vi "N9310A Sweep SR830 Record to file.vi"() -> ()   [LabVIEW 2018]
uses:
  <instrlib>/Stanford Research 830/Public/Data/Read (All Parameters).vi
  <instrlib>/Agilent N9310/Agilent N9310.lvlib
  <instrlib>/Stanford Research 830/Stanford Research 830.lvlib
panel:
  in  "File to save to":path
  out "Measured voltage (V, RMS)":dbl format="%#_6p"
  out "Measured frequency (Hz)":dbl format="%#_6p"
  in  "Input coupling":u16(ring) items=["AC", "DC"]
  in  "Input connection":u16(ring) items=["Single-Ended Voltage", "Differential Voltage", "1 MOhm Current Gain", "100 MOhm Current Gain"]
  in  "Dynamic reserve":i16(ring)=2 items=["High Reserve"=0, "Normal"=1, "Low Noise"=2, "Auto Reserve"=-1]
  in  "Sensitivity":i16(ring)=26 items=["Auto Gain"=-1, "2 nV/fA"=0, "5 nV/fA"=1, "10 nV/fA"=2, "20 nV/fA"=3, "50 nV/fA"=4, "100 nV/fA"=5, "200 nV/fA"=6, "500 nV/fA"=7, "1 uV/pA"=8, "2 uV/pA"=9, "5 uV/pA"=10, "10 uV/pA"=11, "20 uV/pA"=12, "50 uV/pA"=13, "100 uV/pA"=14, "200 uV/pA"=15, "500 uV/pA"=16, "1 mV/nA"=17, "2 mV/nA"=18, "5 mV/nA"=19, "10 mV/nA"=20, "20 mV/nA"=21, "50 mV/nA"=22, "100 mV/nA"=23, "200 mV/nA"=24, "500 mV/mA"=25, "1 V/uA"=26]
  in  "VISA resource name of Stanford SR830":refnum<visa-resource-name>="GPIB0::9::INSTR"
  in  "VISA resource name of Agilent N9310A":refnum<visa-resource-name>="USB0::0x0957::0x2018::01151879::INSTR"
  in  "Wait before measuring (s)":dbl=0.1 format="%#_6p"
  out "Step":dbl format="%^#_6e"
  out "Frequency (Hz)":dbl format="%#_6p"
  in  "Steps":dbl=5.0 format="%^#_6e"
  in  "Amplitude (V)":dbl=0.5 format="%#_6p"
  in  "End frequency (Hz)":dbl=2500.0 format="%#_6p"
  in  "Start frequency (Hz)":dbl=500.0 format="%#_6p"
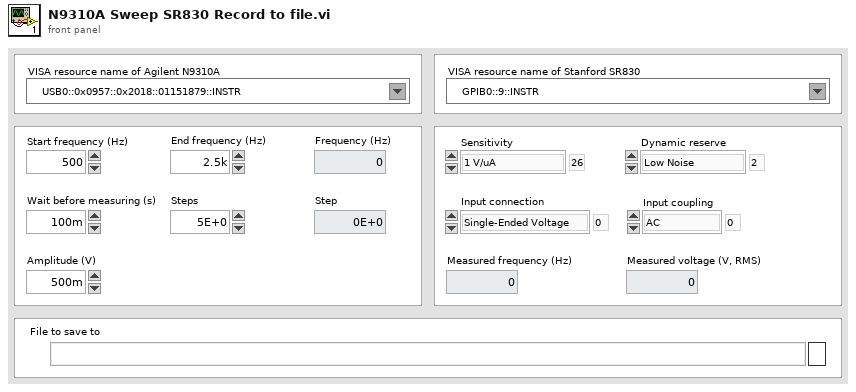
[diagram p1: front panel]
types:
  T1 = cluster{"X-Value":dbl, "Y-Value":dbl, "R-Value":dbl, "Theta-Value":dbl, "Aux In 1 Value":dbl, "Aux In 2 Value":dbl, "Aux In 3 Value":dbl, "Aux In 4 Value":dbl, "Reference Frequency":dbl, "Channel 1 Display":dbl, "Channel 2 Display":dbl}
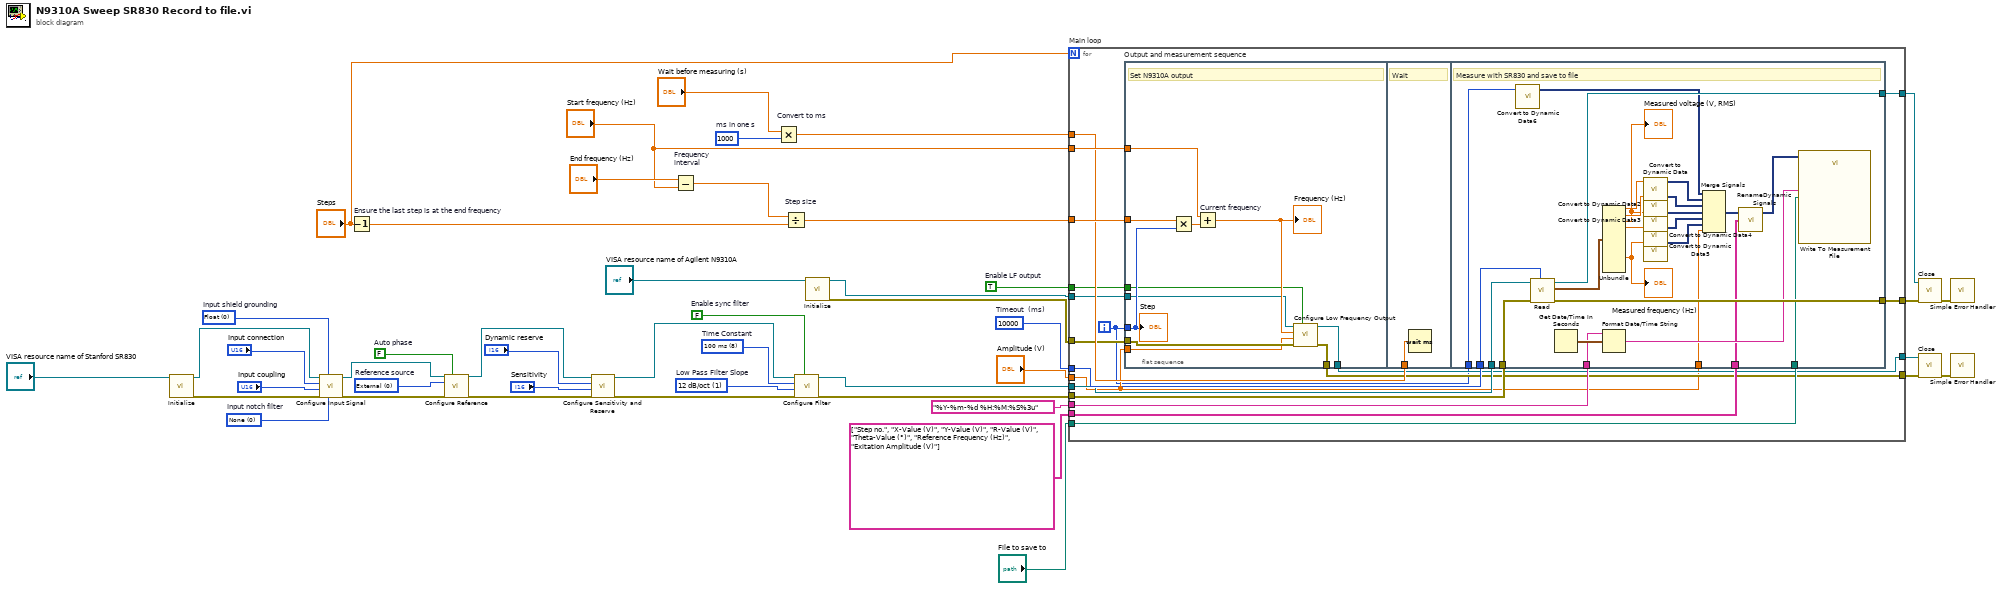
[diagram p0: block diagram]
diagram:
  w9 = u32 10000  # Timeout  (ms)
  w10 = u16 1 items=["6 dB/oct", "12 dB/oct", "18 db/oct", "24 dB/oct"]  # Low Pass Filter Slope
  w11 = u16 8 items=["10 us", "30 us", "100 us", "300 us", "1 ms", "3 ms", "10 ms", "30 ms", "100 ms", "300 ms", "1 s", "3 s", "10 s", "30 s", "100 s", "300 s", "1 ks", "3 ks", "10 ks", "30 ks"]  # Time Constant
  w14 = FALSE  # Enable sync filter
  w19 = FALSE  # Auto phase
  w20 = u16 0 items=["None", "Line Notch", "2x Line Notch", "Both Notch Filters"]  # Input notch filter
  w23 = u16 0 items=["External", "Internal"]  # Reference source
  w27 = u16 0 items=["Float", "Ground"]  # Input shield grounding
  w34 = TRUE  # Enable LF output
  w40 = 1000  # ms in one s
  n1 = call <instrlib>:"Initialize.vi"("VISA resource name"="VISA resource name of Stanford SR830") -> ("error out"=w24:errorcluster, "VISA resource name out"=w28:refnum<visa-resource-name>)  [unwired: 9 in]
  n2 = call <instrlib>:"Configure Input Signal.vi"("Input Notch Filter (0: None)"=w20, "Input Shield Grounding (0: Float)"=w27, "error in (no error)"=w24, "Input Coupling (0: AC)"="Input coupling", "Input Connection (0: Single-Ended Voltage)"="Input connection", "VISA resource name"=w28) -> ("error out"=w21:errorcluster, "VISA resource name out"=w22:refnum<visa-resource-name>)  [unwired: 4 in]
  n3 = Decrement "Ensure the last step is at the end frequency"(x="Steps") -> (x-1=w38:dbl)
  n4 = call <instrlib>:"Configure Reference.vi"("VISA resource name"=w22, "Auto Phase (T: Enabled)"=w19, "Reference Source (1: Internal)"=w23, "error in (no error)"=w21) -> ("VISA resource name out"=w18:refnum<visa-resource-name>, "error out"=w17:errorcluster)  [unwired: 10 in]
  n5 = call <instrlib>:"Configure Sensitivity and Reserve.vi"("error in (no error)"=w17, "Sensitivity (-1: Auto gain)"="Sensitivity", "Dynamic Reserve (-1: Auto Reserve)"="Dynamic reserve", "VISA resource name"=w18) -> ("error out"=w12:errorcluster, "VISA resource name out"=w13:refnum<visa-resource-name>)  [unwired: 6 in]
  n6 = Subtract "Frequency\ninterval"(x="End frequency (Hz)", y="Start frequency (Hz)") -> (x-y=w45:dbl)
  n7 = Multiply "Convert to ms"(x="Wait before measuring (s)", y=w40) -> (x*y=w42:dbl)
  n8 = Divide "Step size"(x=w45, y=w38) -> (x/y=w44:dbl)
  n9 = call <instrlib>:"Configure Filter.vi"("Enable Sync Filter (F: Disable)"=w14, "error in (no error)"=w12, "Low Pass Filter Slope (1: 12dB/oct)"=w10, "Time Constant (8: 100ms)"=w11, "VISA resource name"=w13) -> ("error out"=w7:errorcluster, "VISA resource name out"=w8:refnum<visa-resource-name>)  [unwired: 5 in]
  n10 = call <instrlib>:"Initialize.vi"("VISA resource name"="VISA resource name of Agilent N9310A") -> ("error out"=w35:errorcluster, "VISA resource name out"=w36:refnum<visa-resource-name>)  [unwired: 9 in]
  n11 = for "Main loop" {
    N: "Steps" -> [_]
    tunnel: w44 -> [w64]
    tunnel: "Start frequency (Hz)" -> [w63]
    tunnel: w42 -> [w62]
    tunnel: w36 -> [w51]
    tunnel: w35 -> [w52]
    tunnel: w34 -> [w53]
    tunnel: "Amplitude (V)" -> [w48]
    tunnel: [w49] -> w31
    tunnel: [w50] -> w30
    tunnel: w9 -> [w61]
    tunnel: w8 -> [w60]
    tunnel: w7 -> [w59]
    tunnel: [w58] -> w5
    tunnel: [w57] -> w4
    tunnel: "File to save to" -> [w56]
    tunnel: "%Y-%m-%d %H:%M:%S%3u" -> [w55]
    tunnel: string[] ["Step no.", "X-Value (V)", "Y-Value (V)", "R-Value (V)", "Theta-Value (°)", "Reference Frequency (Hz)", "Exitation Amplitude (V)"] -> [w54]
    i -> [w47]
    n12 = flat-sequence "Output and measurement sequence" {
      tunnel: w47 -> [w71]
      tunnel: w64 -> [w74]
      tunnel: w63 -> [w73]
      tunnel: w53 -> [w70]
      tunnel: w52 -> [w69]
      tunnel: w48 -> [w68]
      tunnel: w51 -> [w67]
      tunnel: [w66] -> w50
      tunnel: [w65] -> w49
      tunnel: w62 -> [w76]
      tunnel: w61 -> [w102]
      tunnel: w60 -> [w101]
      tunnel: w59 -> [w100]
      tunnel: [w99] -> w58
      tunnel: [w98] -> w57
      tunnel: w56 -> [w84]
      tunnel: w55 -> [w83]
      tunnel: w54 -> [w82]
      tunnel: w48 -> [w79]
      tunnel: w47 -> [w78]
      frame #0 {
        # "Set N9310A output"
        n13 = Multiply(x=w74, y=w71) -> (x*y=w75:dbl)
        n14 = Add "Current frequency"(x=w73, y=w75) -> (x+y=w72:dbl)
        "Frequency (Hz)" <- w72
        n15 = call <instrlib>:"Configure Low Frequency Output.vi"("Enable LF Output (F:Disable)"=w70, "error in (no error)"=w69, "Amplitude (0.5 V)"=w68, "Frequency (1.0 kHz)"=w72, "VISA resource name"=w67) -> ("error out"=w66:errorcluster, "VISA resource name out"=w65:refnum<visa-resource-name>)  [unwired: 5 in]
        "Step" <- w71
      }
      frame #1 {
        # "Wait"
        n16 = Wait (ms)(milliseconds to wait=w76) -> ()  [unwired: 1 out]
      }
      frame #2 {
        # "Measure with SR830 and save to file"
        n17 = call "Convert to Dynamic Data6"("Double"=w78) -> ("Dynamic Data Type"=w77:dynamicdata)  [unwired: 3 in]
        n18 = call-poly <instrlib>:"Read.vi"("Timeout (10000 ms)"=w102, "error in (no error)"=w100, "VISA resource name"=w101) -> ("error out"=w98:errorcluster, "Parameter Values"=w86:T1, "VISA resource name out"=w99:refnum<visa-resource-name>)  [unwired: 6 in]
        n19 = Get Date/Time In Seconds() -> (seconds since 1Jan1904=w88:timestamp)
        n20 = Unbundle(w86) -> ("X-Value"=w96:dbl, "Y-Value"=w95:dbl, "R-Value"=w80:dbl, "Theta-Value"=w85:dbl, "Reference Frequency"=w81:dbl)  [unwired: 6 out]
        "Measured frequency (Hz)" <- w81
        "Measured voltage (V, RMS)" <- w80
        n21 = Format Date/Time String(time format string (%c)=w83, seconds (now)=w88) -> (date/time string=w87:string)  [unwired: 1 in]
        n22 = call "Convert to Dynamic Data"("Double"=w96) -> ("Dynamic Data Type"=w89:dynamicdata)  [unwired: 3 in]
        n23 = call "Convert to Dynamic Data2"("Double"=w95) -> ("Dynamic Data Type"=w90:dynamicdata)  [unwired: 3 in]
        n24 = call "Convert to Dynamic Data3"("Double"=w80) -> ("Dynamic Data Type"=w91:dynamicdata)  [unwired: 3 in]
        n25 = call "Convert to Dynamic Data4"("Double"=w85) -> ("Dynamic Data Type"=w92:dynamicdata)  [unwired: 3 in]
        n26 = call "Convert to Dynamic Data5"("Double"=w81) -> ("Dynamic Data Type"=w93:dynamicdata)  [unwired: 3 in]
        n27 = Merge Signals(w77, w89, w90, w91, w92, w93, w79) -> (w94:dynamicdata)
        n28 = call "RenameDynamicSignals.vi"("New Signal Names"=w82, "Dynamic Data In"=w94) -> ("Dynamic Data Out"=w97:dynamicdata)  [unwired: 2 in, 1 out]
        n29 = call "Write To Measurement File"("Signals"=w97, "Filename"=w84, "Comment"=w87) -> ()  [unwired: 14 in, 3 out]
      }
    }
  }
  n30 = call <instrlib>:"Close.vi"("error in (no error)"=w4, "VISA resource name"=w5) -> ("error out"=w6:errorcluster)  [unwired: 9 in]
  n31 = call <instrlib>:"Close.vi"("error in (no error)"=w30, "VISA resource name"=w31) -> ("error out"=w32:errorcluster)  [unwired: 9 in]
  n32 = call <vilib>:"Simple Error Handler.vi"("error in (no error)"=w6) -> ()  [unwired: 4 in, 5 out]
  n33 = call <vilib>:"Simple Error Handler.vi"("error in (no error)"=w32) -> ()  [unwired: 4 in, 5 out]
